vi "_Test_Demo_example.vi"() -> ()   [LabVIEW 2023]
uses:
  DSLV_Tree/DSLV_Tree.lvlib
panel:
  in  "Tab Control":T1(tab)
  in  "Tri-State?":bool=TRUE
  out "Seted Tags":T2(array[cluster])
  out "Children Tags":string[](array[string])
  out "Selected?":bool[](array[boolean])
  in  "Test Get children":bool=TRUE
  in  "pure children？":bool
  in  "Change":bool
  in  "Status":string(combo)
  out "error out":errorcluster
  in  "Tree":string(tree)
  # "RUN THIS VI AND CHOSE ONE TAB FOR YOUR FUNCTION TEST NEED"
  # "Test1 - Tree Selection\n*press the tree checkbox,you can see the changed status of the Nodes releated\n*you can right-click the tree tag to change all the tree checkbox\n*optional - enable/disable Tri-State then the status of the checkbox would some different"
  # "Test2 - Check Checkbox\n*press the Test Get children to got the bool array if the Tree Tag is selected.\n*optional - enable/disable pure children button, then the output of the array exclude/include the section node."
  # "Test3 - Change Status\n*press the tree to selection a tag depend to change status\n*select a desired status via pull down the Status control\n*press the Change button then you can see the changes"
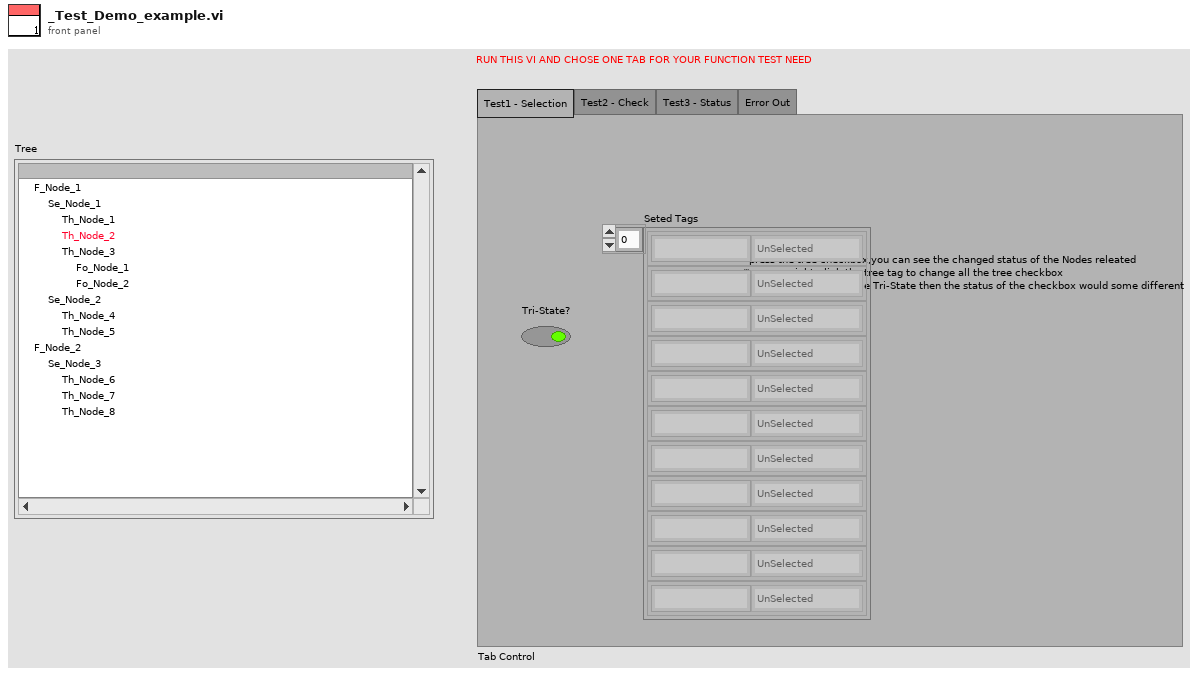
[diagram p1: front panel]
types:
  T1 = enum32{"Test1 - Selection", "Test2 - Check", "Test3 - Status", "Error Out"}
  T2 = cluster{"Tag":string, "Selected?":enum16{"UnSelected", "Selected", "PartSelected"}}[]
  T3 = typedef "LVPoint32TypeDef.ctl" = cluster{"Horizontal":i32, "Vertical":i32}
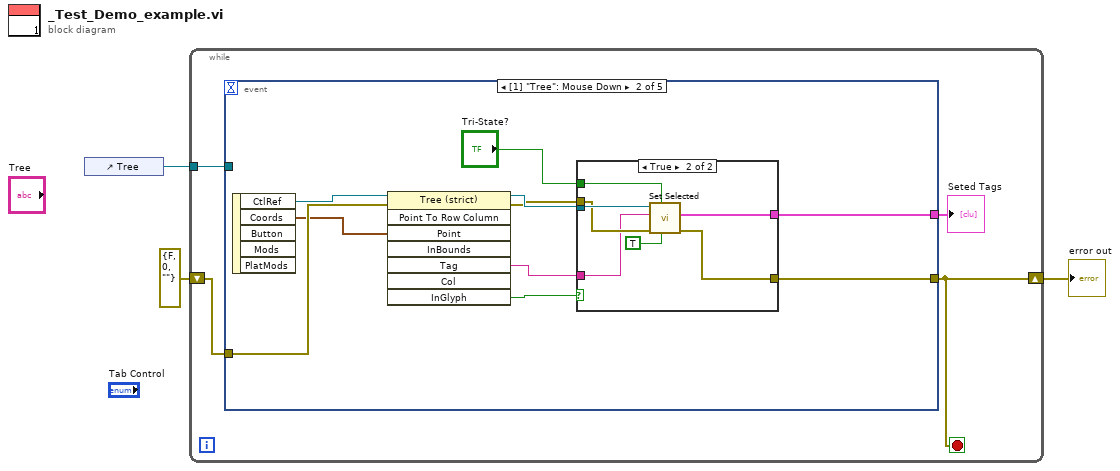
[diagram p0: block diagram]
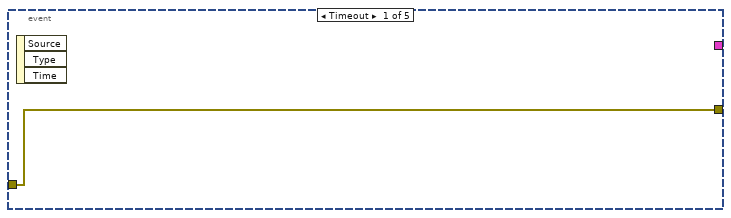
[diagram p2: hidden frame]
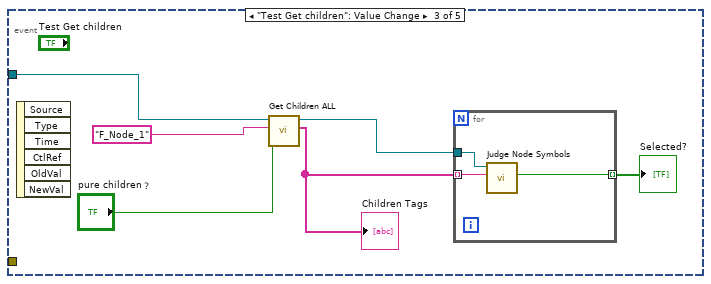
[diagram p4: hidden frame]
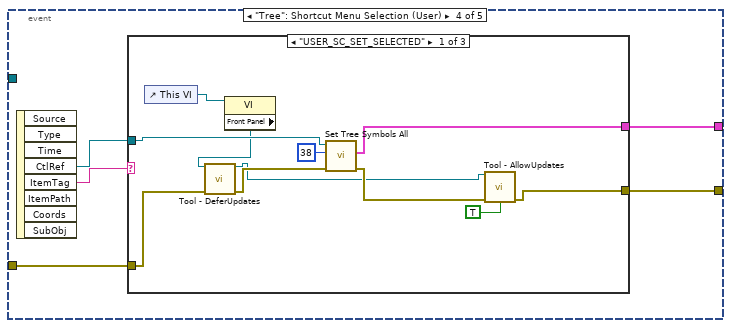
[diagram p5: hidden frame]
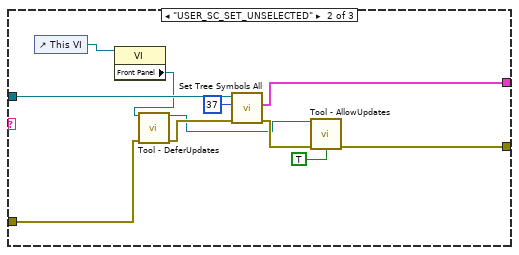
[diagram p6: hidden frame]
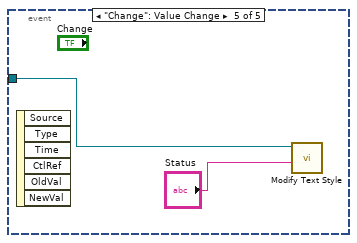
[diagram p8: hidden frame]
diagram:
  n1 = control-ref of="Tree"() -> (w1:refnum<vi>)
  n2 = while {
    shift-right: [w6] -> w3
    shift-left: errorcluster {"status"=FALSE, "code"=0, "source"=""} ("error out") -> [w7]
    tunnel: w1 -> [w4]
    stop <- w6 stop-if-true
    n3 = event shown="[1] \"Tree\": Mouse Down" {
      selector: _ -> [_ _ _ _ _]
      dyn-events: _ -> [_ _ _ _ _]
      timeout: _ -> [_ _ _ _ _]
      tunnel: [w8 w18 _ w38 _] -> w6
      tunnel: w7 -> [w8 w14 _ w37 _]
      tunnel: [_ w17 _ w36 _] -> w5
      tunnel: w4 -> [_ _ w32 _ w64]
      event Timeout {
        n4 = event-data() -> ()  [unwired: 1 in, 3 out]
      }
      event "Tree": Mouse Down {
        n5 = event-data() -> ("CtlRef"=w16:refnum<vi>, "Coords"=w12:T3)  [unwired: 1 in, 3 out]
        n6 = invoke on="Invoke Node" class="Tree (strict)" method="Point To Row Column"(reference=w16, error in=w14, "Point"=w12) -> (reference out=w15:refnum<vi>, error out=w13:errorcluster, "Tag"=w10:string, "InGlyph"=w11:bool)  [unwired: 5 in, 4 out]
        n7 = case shown="True" w11 {
          tunnel: [w19 w26] -> w18
          tunnel: [_ w25] -> w17
          tunnel: w15 -> [_ w24]
          tunnel: w13 -> [w19 w23]
          tunnel: w10 -> [_ w21]
          tunnel: "Tri-State?" -> [_ w20]
          frame False {
          }
          frame True {
            n8 = call "Set Selected.vi"("Get All Children?"=TRUE, "Tri-State?"=w20, "error in (no error)"=w23, "Tag"=w21, "Tree Reference"=w24) -> ("error out"=w26:errorcluster, "Seted Tags"=w25:T2)  [unwired: 4 in, 1 out]
          }
        }
      }
      event "Test Get children": Value Change {
        n9 = event-data() -> ()  [unwired: 1 in, 6 out]
        n10 = call "Get Children ALL.vi"("pure children？"="pure children？", "Parent Tag"="F_Node_1", "Tree Reference"=w32) -> ("Children Tags"=w29:string[], "Tree Reference"=w28:refnum<vi>)  [unwired: 6 in, 1 out]
        "Children Tags" <- w29
        n11 = for {
          tunnel: w29 -> [w35] mode=indexing
          tunnel: w28 -> [w34]
          tunnel: [w33] -> w27 mode=indexing
          n12 = call "Judge Node Symbols.vi"("Tag"=w35, "TreeControl in"=w34) -> ("Selected?"=w33:bool)  [unwired: 7 in, 2 out]
        }
        "Selected?" <- w27
      }
      event "Tree": Shortcut Menu Selection (User) {
        n13 = event-data() -> ("CtlRef"=w39:refnum<vi>, "ItemTag"=w40:string)  [unwired: 1 in, 6 out]
        n14 = case shown="\"USER_SC_SET_SELECTED\"" w40 {
          tunnel: w39 -> [w50 w62 _]
          tunnel: [w43 w54 w63] -> w38
          tunnel: w37 -> [w42 w53 w63]
          tunnel: [w41 w52 _] -> w36
          frame "USER_SC_SET_SELECTED" {
            n15 = control-ref of="This VI"() -> (w49:refnum<vi>)
            n16 = property class="VI"(reference=w49) -> ("Front Panel"=w48:refnum<vi>)  [unwired: 1 in, 2 out]
            n17 = call "Tool - DeferUpdates.vi"("Panel Ref In"=w48, "error in (no error)"=w42) -> ("Panel Ref Out"=w45:refnum<vi>, "error out"=w47:errorcluster)  [unwired: 12 in]
            n18 = call "Set Tree Symbols All.vi"("error in (no error)"=w47, "symbol"=38, "Tree Refnum"=w50) -> ("error out"=w46:errorcluster, "Seted Tags"=w41:T2)  [unwired: 6 in, 1 out]
            n19 = call "Tool - AllowUpdates.vi"("Panel ref in"=w45, "error in (no error)"=w46, "Clear Ref? (F)"=TRUE) -> ("error out"=w43:errorcluster)  [unwired: 11 in, 1 out]
          }
          frame "USER_SC_SET_UNSELECTED" {
            n20 = control-ref of="This VI"() -> (w60:refnum<vi>)
            n21 = property class="VI"(reference=w60) -> ("Front Panel"=w57:refnum<vi>)  [unwired: 1 in, 2 out]
            n22 = call "Tool - DeferUpdates.vi"("Panel Ref In"=w57, "error in (no error)"=w53) -> ("Panel Ref Out"=w56:refnum<vi>, "error out"=w59:errorcluster)  [unwired: 12 in]
            n23 = call "Set Tree Symbols All.vi"("error in (no error)"=w59, "symbol"=37, "Tree Refnum"=w62) -> ("error out"=w58:errorcluster, "Seted Tags"=w52:T2)  [unwired: 6 in, 1 out]
            n24 = call "Tool - AllowUpdates.vi"("Panel ref in"=w56, "error in (no error)"=w58, "Clear Ref? (F)"=TRUE) -> ("error out"=w54:errorcluster)  [unwired: 11 in, 1 out]
          }
          frame Default {
          }
        }
      }
      event "Change": Value Change {
        n25 = event-data() -> ()  [unwired: 1 in, 6 out]
        n26 = call "Modify Text Style.vi"("Status"="Status", "Tree Reference"=w64) -> ()  [unwired: 8 in, 2 out]
      }
    }
    "Seted Tags" <- w5
  }
  "error out" <- w3
